vi "CloseDialog.vi"() -> (3 "Which Button?":T1(ring)=enum."Center Button")   [LabVIEW 2016]
doc: "Displays text in a dialog with three buttons. The output enum indicates which of the three buttons the user chose, or it indicates that the user closed the dialog without making any choice."
panel:
  in  "Board":bool
  in  "Right Button":bool
  in  "Center Button":bool
  in  "Left Button":bool
  # "Do you want to update your program?"
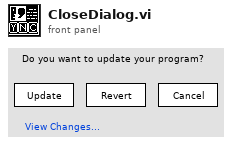
[diagram p1: front panel]
types:
  T1 = enum16{"Left Button", "Center Button", "Right Button", "Window Close"}
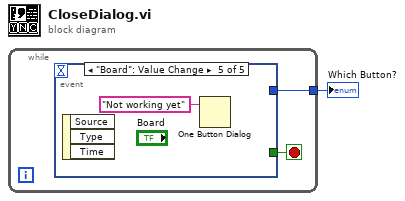
[diagram p0: block diagram]
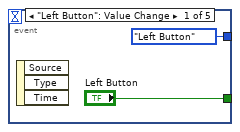
[diagram p2: hidden frame]
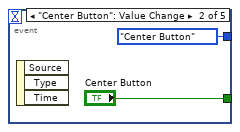
[diagram p3: hidden frame]
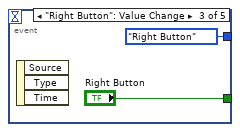
[diagram p4: hidden frame]
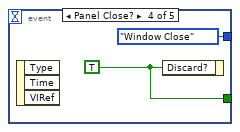
[diagram p5: hidden frame]
diagram:
  n1 = while {
    tunnel: [w3] -> w1
    stop <- w2 stop-if-true
    n2 = event shown="[4] \"Board\": Value Change" {
      selector: _ -> [_ _ _ _ _]
      dyn-events: _ -> [_ _ _ _ _]
      timeout: _ -> [_ _ _ _ _]
      tunnel: ["Left Button" "Center Button" "Right Button" w10 _] -> w2
      tunnel: [T1."Left Button" ("Which Button?") T1."Center Button" ("Which Button?") T1."Right Button" ("Which Button?") T1."Window Close" ("Which Button?") _] -> w3
      event "Left Button": Value Change {
        n3 = event-data() -> ()  [unwired: 1 in, 3 out]
      }
      event "Center Button": Value Change {
        n4 = event-data() -> ()  [unwired: 1 in, 3 out]
      }
      event "Right Button": Value Change {
        n5 = event-data() -> ()  [unwired: 1 in, 3 out]
      }
      event Panel Close? {
        w10 = TRUE ("Discard?")
        n6 = event-data() -> ()  [unwired: 1 in, 3 out]
        n7 = event-data("Discard?"=w10) -> ()  [unwired: 1 in, 1 out]
      }
      event "Board": Value Change {
        n8 = event-data() -> ()  [unwired: 1 in, 3 out]
        n9 = One Button Dialog(message="Not working yet") -> ()  [unwired: 1 in, 1 out]
      }
    }
  }
  "Which Button?" <- w1
